vi "table重新排序.vi"(11 "tables":string[](array[string])) -> (3 "sorted elements":string[](array[string]))   [LabVIEW 2016, in "数据查询.lvlib"]
uses:
  <userlib>/_OpenG.lib/array/array.llb/Delete Elements from 1D Array (String)__ogtk.vi
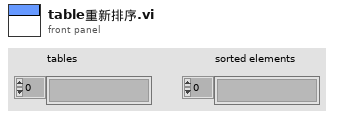
[diagram p1: front panel]
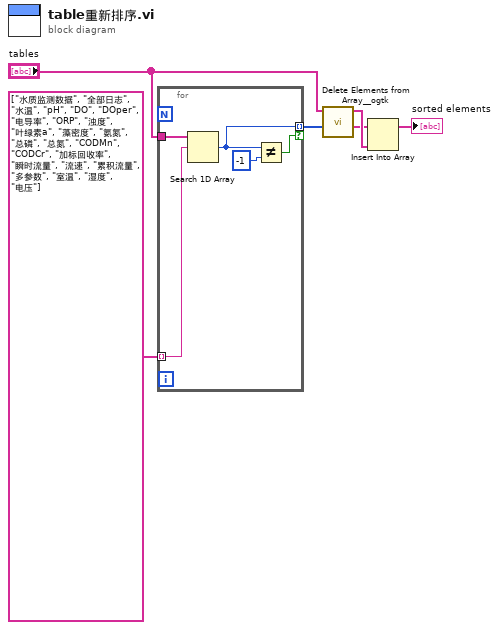
[diagram p0: block diagram]
diagram:
  n1 = for {
    tunnel: "tables" -> [w9]
    tunnel: string[] ["水质监测数据", "全部日志", "水温", "pH", "DO", "DOper", "电导率", "ORP", "浊度", "叶绿素a", "藻密度", "氨氮", "总磷", "总氮", "CODMn", "CODCr", "加标回收率", "瞬时流量", "流速", "累积流量", "多参数", "室温", "湿度", "电压"] ("tables") -> [w11] mode=indexing
    tunnel: [w8] -> w4 mode=indexing if=w7
    n2 = Search 1D Array(1D array=w9, element=w11) -> (index of element=w8:i32)  [unwired: 1 in]
    n3 = Not Equal?(x=w8, y=-1) -> (x != y?=w7:bool)
  }
  n4 = call-poly <userlib>:"Delete Elements from Array__ogtk.vi"("indices"=w4, "array"="tables") -> ("deleted elements"=w5:string[], "array w/ subset deleted"=w6:string[])  [unwired: 8 in]
  n5 = Insert Into Array(array=w5, new element=w6) -> (→"sorted elements":string[])  [unwired: 1 in]
